vi "Periodic Tasks.vi"(8 "error in":errorcluster) -> ()   [LabVIEW 2017]
doc: "This VI runs in parallel to other robot code. It can contain as many user-defined periodic loops as you need. These can carry out PID or other sorts of timed response."
uses:
  <vilib>/Rock Robotics/WPI/Utilities/WPI_GetSetVariantRefNum.vi
  <vilib>/ptbypt/NI_PtbyPt.lvlib
  Support Code/TipWarning.vi
panel:
  in  "threshold":dbl(slide)=10.0 min=10.0 max=20.0 scale=10.0..20.0
  out "Waveform Chart":cluster{dbl, i16}(graph)
  in  "sample length":i32=100
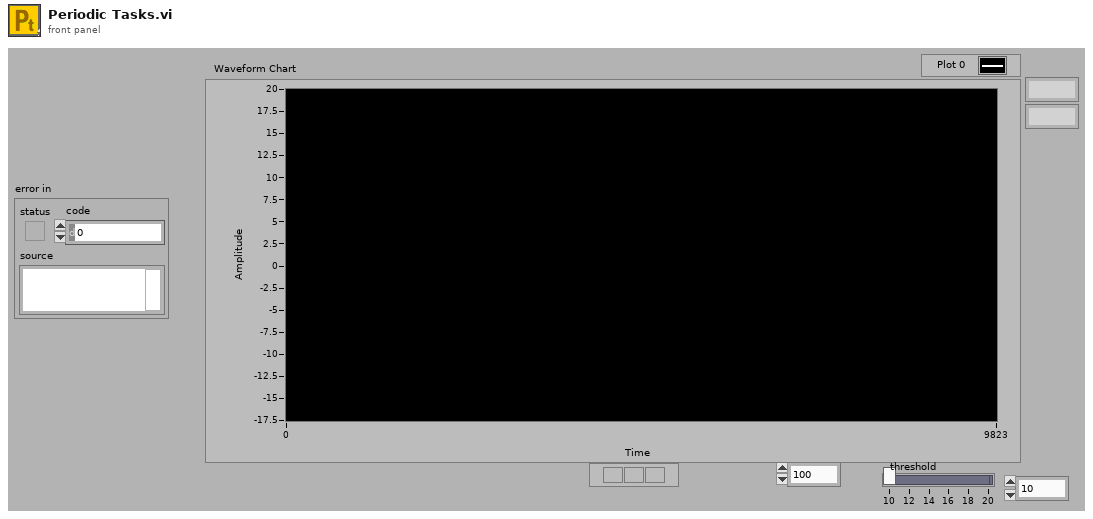
[diagram p1: front panel]
types:
  T1 = typedef "WPI_AccelerometerDevRef.ctl" = cluster{"DevStatus":errorcluster, "Scaling":T2, "Analog Channels":T3, "I2C Bus":T5, "SPI Bus":T6, "Accel Range":T7, "ADXL Axes":T8, "Handle":i32, "Device Address":u8, "Accel Type":enum16{"Analog", "ADXL345 I2C", "ADXL345 SPI", "Internal", "ADXL362 SPI"}}
  T2 = typedef "WPI_AccelerometerScaling.ctl" = cluster{"Gain (VoltsPerG)":dbl, "Center Voltage":dbl}
  T3 = typedef "WPI_AccelerometerAnalogChannels.ctl" = cluster{"X-Axis":T4, "Y-Axis":T4, "Z-Axis":T4}
  T4 = typedef "FPGA_AIChannel.ctl" = enum8{"AI 0", "AI 1", "AI 2", "AI 3", "AI MXP 0", "AI MXP 1", "AI MXP 2", "AI MXP 3", "Invalid"}
  T5 = typedef "i2c_bus.ctl" = enum16{"I2C On-Board", "I2C MXP", "Invalid"}
  T6 = typedef "spi_bus.ctl" = enum16{"SPI On-Board, CS0", "SPI On-Board, CS1", "SPI On-Board, CS2", "SPI On-Board, CS3", "SPI MXP", "Invalid"}
  T7 = typedef "ADXL345 Range.ctl" = u8
  T8 = typedef "WPI_AccelerometerADXL345 Axes.ctl" = cluster{"X-Axis":bool, "Y-Axis":bool, "Z-Axis":bool}
  T9 = cluster{"X-Axis":dbl, "Y-Axis":dbl, "Z-Axis":dbl}
  T10 = typedef "WPI_JoystickDevRef.ctl" = cluster{"Device":T11}
  T11 = typedef "WPI_JoystickDeviceEnum.ctl" = enum16{"USB 0", "USB 1", "USB 2", "USB 3", "USB 4", "USB 5"}
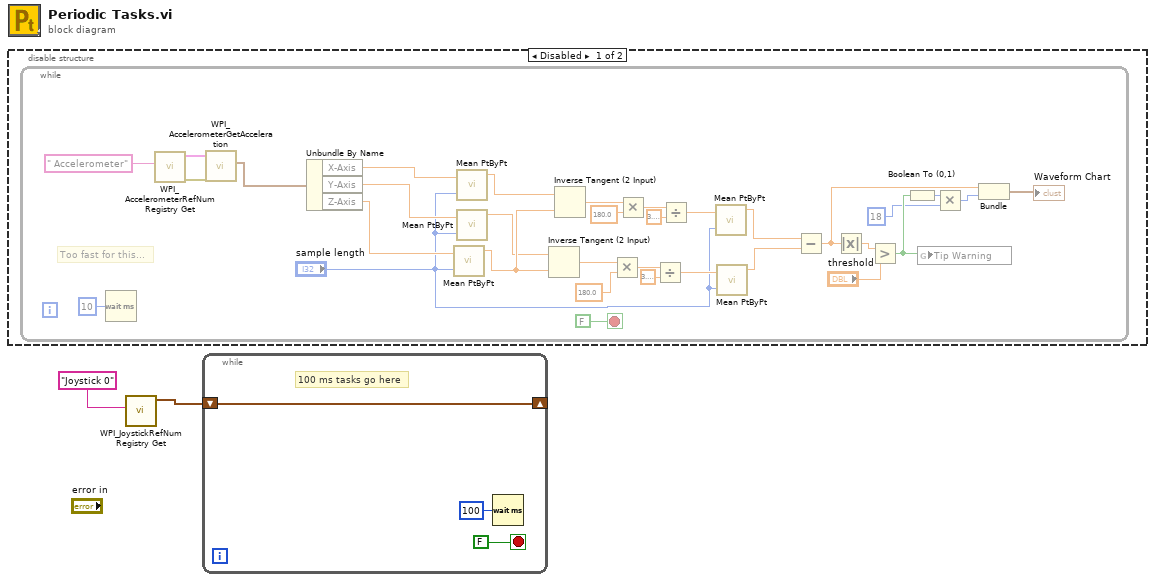
[diagram p0: block diagram]
diagram:
  n1 = disable-structure shown="Disabled" {
    frame Disabled {
      n2 = while {
        stop <- FALSE stop-if-true
        # "Too fast for this..."
        n3 = Wait (ms)(milliseconds to wait=u32 10) -> ()  [unwired: 1 out]
        n4 = call <vilib>:"WPI_AccelerometerRefNum Registry Get.vi"("refnum name"=" Accelerometer") -> ("error out"=w35:errorcluster, "AccelerometerDevRef"=w34:T1)  [unwired: 9 in]
        n5 = call <vilib>:"WPI_AccelerometerGetAcceleration.vi"("error in"=w35, "AccelerometerDevRef"=w34) -> ("Accelerations"=w33:T9)  [unwired: 7 in, 2 out]
        n6 = Unbundle By Name(w33) -> ("X-Axis"=w13:dbl, "Y-Axis"=w28:dbl, "Z-Axis"=w29:dbl)
        n7 = call <vilib>:"Mean PtByPt.vi"("x"=w29, "sample length"="sample length") -> ("mean"=w20:dbl)  [unwired: 2 in, 1 out]
        n8 = call <vilib>:"Mean PtByPt.vi"("x"=w13, "sample length"="sample length") -> ("mean"=w19:dbl)  [unwired: 2 in, 1 out]
        n9 = call <vilib>:"Mean PtByPt.vi"("x"=w28, "sample length"="sample length") -> ("mean"=w18:dbl)  [unwired: 2 in, 1 out]
        n10 = Inverse Tangent (2 Input)(1:w20, 2:w18) -> (0:w17:dbl)
        n11 = Inverse Tangent (2 Input)(1:w20, 2:w19) -> (0:w24:dbl)
        n12 = Multiply(x=w17, y=180.0) -> (x*y=w22:dbl)
        n13 = Multiply(x=w24, y=180.0) -> (x*y=w26:dbl)
        n14 = Divide(x=w22, y=3.141592653589793) -> (x/y=w16:dbl)
        n15 = Divide(x=w26, y=3.141592653589793) -> (x/y=w15:dbl)
        n16 = call <vilib>:"Mean PtByPt.vi"("x"=w15, "sample length"="sample length") -> ("mean"=w11:dbl)  [unwired: 2 in, 1 out]
        n17 = call <vilib>:"Mean PtByPt.vi"("x"=w16, "sample length"="sample length") -> ("mean"=w12:dbl)  [unwired: 2 in, 1 out]
        n18 = Subtract(x=w11, y=w12) -> (x-y=w9:dbl)
        n19 = Absolute Value(x=w9) -> (abs(x)=w10:dbl)
        n20 = Greater?(x=w10, y="threshold") -> (0:w8:bool)
        n21 = Boolean To (0,1)(Boolean=w8) -> (0, 1=w6:i16)
        n22 = global write "TipWarning.vi" "Tip Warning"(w8) -> ()
        n23 = Multiply(x=w6, y=i16 18) -> (x*y=w5:i16)
        n24 = Bundle(w9, w5) -> (→"Waveform Chart":cluster{dbl, i16})  [unwired: 1 in]
      }
    }
    frame Enabled {
    }
  }
  n25 = call <vilib>:"WPI_JoystickRefNum Registry Get.vi"("refnum name"="Joystick 0") -> ("JoystickDevRef"=w1:T10)  [unwired: 1 in, 9 out]
  n26 = while {
    shift-right: [w36] -> _
    shift-left: w1 -> [w36]
    stop <- FALSE stop-if-true
    # "100 ms tasks go here"
    n27 = Wait (ms)(milliseconds to wait=u32 100) -> ()  [unwired: 1 out]
  }
